vi "获取帮助文档.vi"   [LabVIEW 2019]
uses:
  <vilib>/Platform/browser.llb/Open URL in Default Browser (path).vi
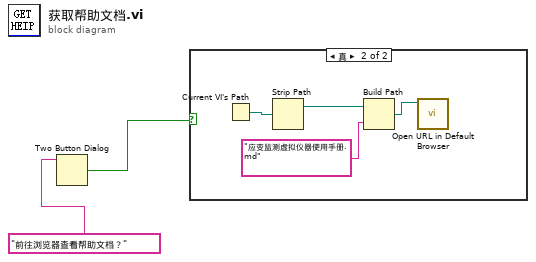
[diagram p0: block diagram]
diagram:
  n1 = Two Button Dialog(message="前往浏览器查看帮助文档？" ("消息")) -> (T button?=w1:bool)  [unwired: 2 in]
  n2 = case shown="真" w1 {
    frame False {
    }
    frame True {
      n3 = Current VI's Path() -> (path=w5:path)
      n4 = Strip Path(path=w5) -> (stripped path=w3:path)  [unwired: 1 out]
      n5 = Build Path(base path=w3, name or relative path="应变监测虚拟仪器使用手册.md") -> (appended path=w4:path)
      n6 = call-poly <vilib>:"Open URL in Default Browser.vi"("path"=w4) -> ()  [unwired: 5 in, 2 out]
    }
  }
